vi "fullConstructor.vi"(10 "Size":u32, 11 "Key-Value Pairs":T1[](array[typedef])) -> (0 "error out":errorcluster, 3 "Bucket out":refnum<class "Bucket.lvclass">)   [LabVIEW 2017, in "Bucket.lvclass"]
uses:
  <userlib>/836-Library/Data_Structures/Bucket/Bucket.lvclass
  <userlib>/836-Library/Data_Structures/Bucket/Types/KeyValuePair.ctl
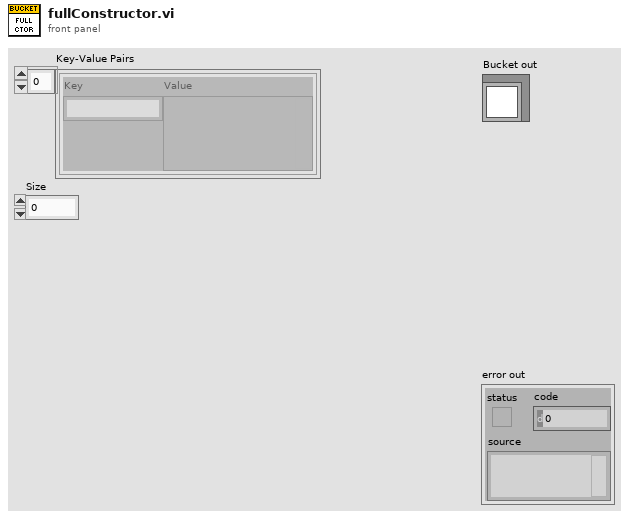
[diagram p1: front panel]
types:
  T1 = typedef "KeyValuePair.ctl" = cluster{"Key":string, "Value":variant}
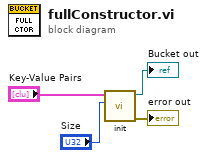
[diagram p0: block diagram]
diagram:
  n1 = call <userlib>:"init.vi"("Size"="Size", "Key Value Pairs"="Key-Value Pairs") -> ("error out"=→"error out":errorcluster, "Bucket out"=→"Bucket out":refnum<class "Bucket.lvclass">)  [unwired: 8 in]
